vi "Configure Current Limit.vi"(6 "behavior (regulate)":i32(ring) items=["Regulate", "Trip"], 8 "error in (no error)":errorcluster, 9 "limit (0.0 Amps)":dbl[unit] format="%^.2e", 10 "channel name (\"CHANNEL1\")":string="CHANNEL1", 11 "CS++DCPwr in":refnum<class "CS++DCPwr.lvclass">) -> (0 "error out":errorcluster, 3 "CS++DCPwr out":refnum<class "CS++DCPwr.lvclass">)   [LabVIEW 2013, in "CS++DCPwr.lvlib" / "CS++DCPwr.lvclass"]
doc: "This VI configures the current limit. You specify the output current limit value and the behavior of the power supply when the output current is greater than or equal to that value."
uses:
  CS++DCPwr.lvclass
  CSPP_Core/Classes/CS++ProcessVariables/ProcessVariable/PV.lvclass
  CS++DCPwr.lvclass/CS++DCPwr.ctl
  CSPP_Core/Classes/CS++ProcessVariables/PVConnection/PVConnection.lvclass
  CSPP_Core/Classes/CS++ProcessVariables/ProcessVariable/PV.lvclass/PV.ctl
  CSPP_Core/Classes/CS++ProcessVariables/ProcessVariable/Write Data.vi
  CSPP_Core/Classes/CS++ProcessVariables/ProcessVariable/Write Timestamp.vi
  CSPP_Core/Classes/CS++ProcessVariables/ProcessVariable/Write Quality.vi
  CSPP_Core/Classes/CS++ProcessVariables/ProcessVariable/Write status.vi
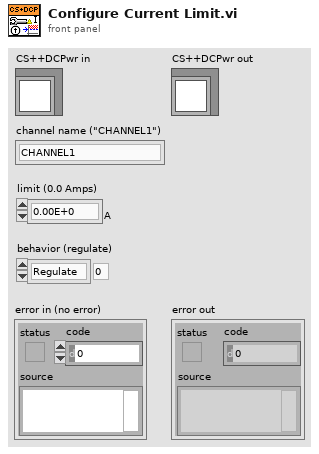
[diagram p1: front panel]
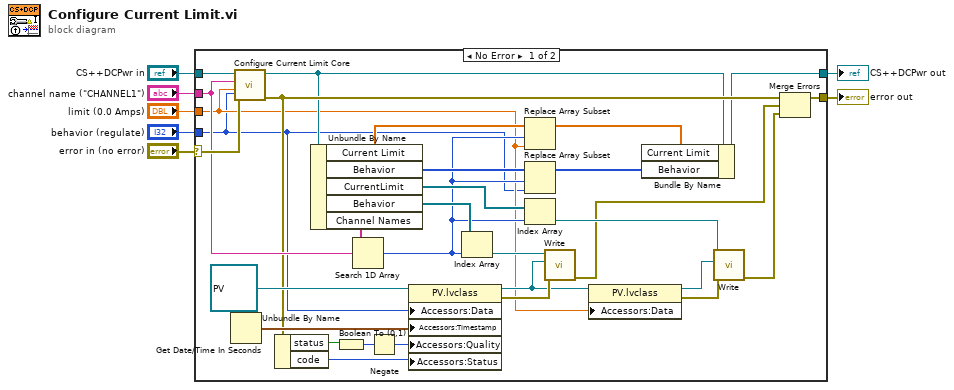
[diagram p0: block diagram]
diagram:
  n1 = case shown="No Error" "error in (no error)" {
    selector: "error in (no error)" -> [w37 w40]
    tunnel: [w29 w40] -> w5
    tunnel: [w20 w39] -> w6
    tunnel: "CS++DCPwr in" -> [w38 w39]
    tunnel: "channel name (\"CHANNEL1\")" -> [w32 _]
    tunnel: "behavior (regulate)" -> [w8 _]
    tunnel: "limit (0.0 Amps)" -> [w9 _]
    frame No Error {
      n2 = Get Date/Time In Seconds() -> (seconds since 1Jan1904=w36:timestamp)
      n3 = call-dynamic "Configure Current Limit Core.vi"("behavior (regulate)"=w8, "error in (no error)"=w37, "limit (0.0 Amps)"=w9, "channel name (\"CHANNEL1\")"=w32, "CS++DCPwr in"=w38) -> ("error out"=w24:errorcluster, "CS++DCPwr out"=w21:refnum<class "CS++DCPwr.lvclass">)  [unwired: 5 in]
      n4 = Unbundle By Name(w24) -> ("status"=w28:bool, "code"=w26:i32)
      n5 = Unbundle By Name(w21) -> ("Current Limit"=w19:dbl[unit][], "Behavior"=w23:i32[], "CurrentLimit"=w14:refnum<class "PVConnection.lvclass">[], "Behavior"=w31:refnum<class "PVConnection.lvclass">[], "Channel Names"=w33:string[])
      n6 = Boolean To (0,1)(Boolean=w28) -> (0, 1=w27:i16)
      n7 = Search 1D Array(1D array=w33, element=w32) -> (index of element=w13:i32)  [unwired: 1 in]
      n8 = Negate(x=w27) -> (-x=w25:i16)
      n9 = property class="PV.lvclass"(reference=refnum<class "PV.lvclass"> refnum ("PV"), "Accessors:Data"=w8, "Accessors:Timestamp"=w36, "Accessors:Quality"=w25, "Accessors:Status"=w26) -> (reference out=w12:refnum<class "PV.lvclass">, error out=w34:errorcluster)  [unwired: 1 in]
      n10 = Index Array(array=w31, index=w13) -> (element=w30:refnum<class "PVConnection.lvclass">)
      n11 = Replace Array Subset(array=w19, new element=w9, index=w13) -> (w18:dbl[unit][])
      n12 = Replace Array Subset(array=w23, new element=w8, index=w13) -> (w22:i32[])
      n13 = Index Array(array=w14, index=w13) -> (element=w17:refnum<class "PVConnection.lvclass">)
      n14 = call-dynamic "Write.vi"("error in (no error)"=w34, "PV"=w12, "PVConnection in"=w30) -> ("error out"=w11:errorcluster)  [unwired: 7 in, 1 out]
      n15 = property class="PV.lvclass"(reference=w12, "Accessors:Data"=w9) -> (reference out=w16:refnum<class "PV.lvclass">, error out=w15:errorcluster)  [unwired: 1 in]
      n16 = Bundle By Name(cluster=w21, "Current Limit"=w18, "Behavior"=w22) -> (w20:refnum<class "CS++DCPwr.lvclass">)
      n17 = call-dynamic "Write.vi"("error in (no error)"=w15, "PV"=w16, "PVConnection in"=w17) -> ("error out"=w10:errorcluster)  [unwired: 7 in, 1 out]
      n18 = Merge Errors(w24, w11, w10) -> (w29:errorcluster)
    }
    frame Error {
    }
  }
  "error out" <- w5
  "CS++DCPwr out" <- w6
